vi "TEST_Exec State.vi"() -> ()   [LabVIEW 2009]
panel:
  in  "stop":bool
  out "resulting string":string
  out "error out":errorcluster
  in  "error in (no error)":errorcluster
  in  "SRV In":refnum<k5>
  in  "Sensors Config File Path":path=path "C:/SRV/Config/mike_SensorsConfig.xml"
  out "VI refnum out":refnum<vi>
  in  "VI Path":path=path "C:/SRV/SRV VIs/Sensors/SRV_Sensor View Tab GUI.vi"
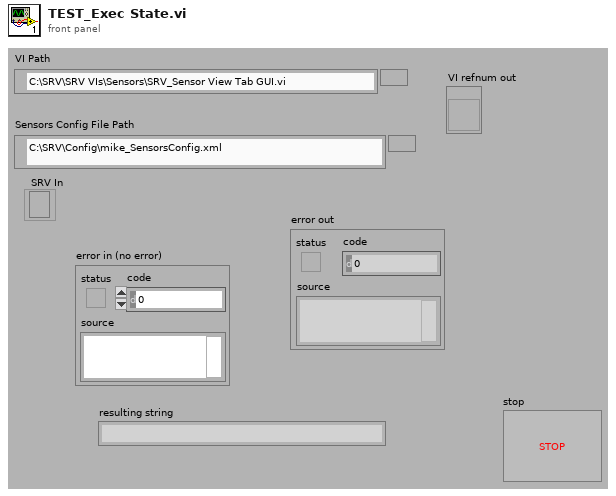
[diagram p1: front panel]
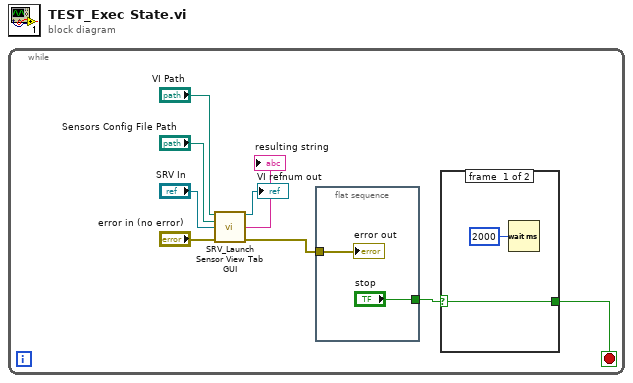
[diagram p0: block diagram]
diagram:
  n1 = while {
    stop <- w1 stop-if-true
    n2 = call "SRV_Launch Sensor View Tab GUI.vi"("VI Path"="VI Path", "Sensors Config File Path"="Sensors Config File Path", "SRV In"="SRV In", "error in (no error)"="error in (no error)") -> ("VI refnum out"=→"VI refnum out":refnum<vi>, "resulting string"=→"resulting string":string, "error out"=w4:errorcluster)  [unwired: 9 in]
    n3 = flat-sequence {
      tunnel: w4 -> [w14]
      tunnel: ["stop"] -> w2
      frame #0 {
        "error out" <- w14
      }
    }
    n4 = case shown="False" w2 {
      selector: w2 -> [w11 w12]
      tunnel: [w11 w12] -> w1
      frame #0 {
        n5 = Wait (ms)(milliseconds to wait=u32 2000) -> ()  [unwired: 1 out]
      }
      frame #1 {
      }
    }
  }
